vi "GenNet-Client Report Error.vi"(6 "Caller MsgQ":refnum<class "DQMH-GenNet Message Queue.lvclass">, 8 "error in":errorcluster) -> (0 "error out":errorcluster)   [LabVIEW 2014, in "GenNet-Client.lvlib"]
doc: "If <b>error in</b> is true, sends the error cluster to the caller's Error case in the MHL through the <b>Caller MsgQ</b>"
uses:
  GenNet-Client.lvlib
  DQMH-GenNet Message Queue.lvclass
  <vilib>/Delacor/Delacor QMH/Libraries/Message Queue_class/Delacor_lib_QMH_Message Queue.lvclass/Delacor_lib_QMH_Message Queue.ctl
  <vilib>/Delacor/Delacor QMH/Libraries/Message Queue_class/Delacor_lib_QMH_Enqueue Message (Single).vi
  <vilib>/Delacor/Delacor QMH/Libraries/Message Queue_class/Delacor_lib_QMH_Message Queue.lvclass
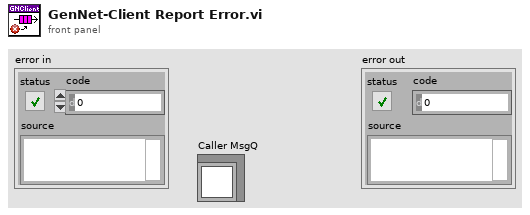
[diagram p1: front panel]
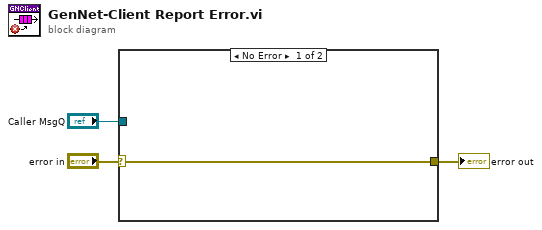
[diagram p0: block diagram]
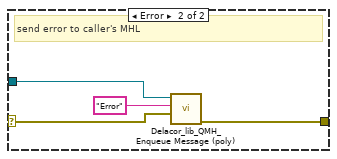
[diagram p2: hidden frame]
diagram:
  n1 = case shown="No Error" "error in" {
    selector: "error in" -> [w4 w5]
    tunnel: "Caller MsgQ" -> [_ w7]
    tunnel: [w4 w6] -> w2
    frame No Error {
    }
    frame Error {
      # "send error to caller's MHL"
      n2 = call-poly <vilib>:"Delacor_lib_QMH_Enqueue Message (poly).vi"("Message Data"=w5, "Message"="Error", "Message Queue in"=w7) -> ("error out"=w6:errorcluster)  [unwired: 7 in, 1 out]
    }
  }
  "error out" <- w2
